vi "sTRING.vi"(6 "angulo":dbl, 8 "Valor del voltaje":dbl, 9 "cadena entrada":string, 10 "Orden":T1(array[ring]), 11 "arreglo opciones":bool[](array[boolean])=[FALSE, FALSE, FALSE, FALSE]) -> (2 "String":string)   [LabVIEW 2016]
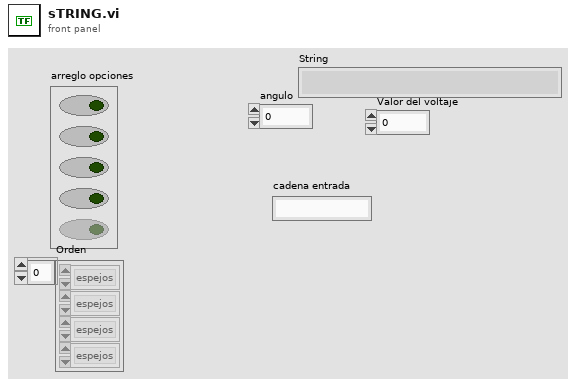
[diagram p1: front panel]
types:
  T1 = enum16{"espejos", "polarizador", "voltaje", "potenciometro y lockin", "CCD"}[]
  T2 = enum16{"espejos", "polarizador", "voltaje", "potenciometro y lockin", "CCD"}
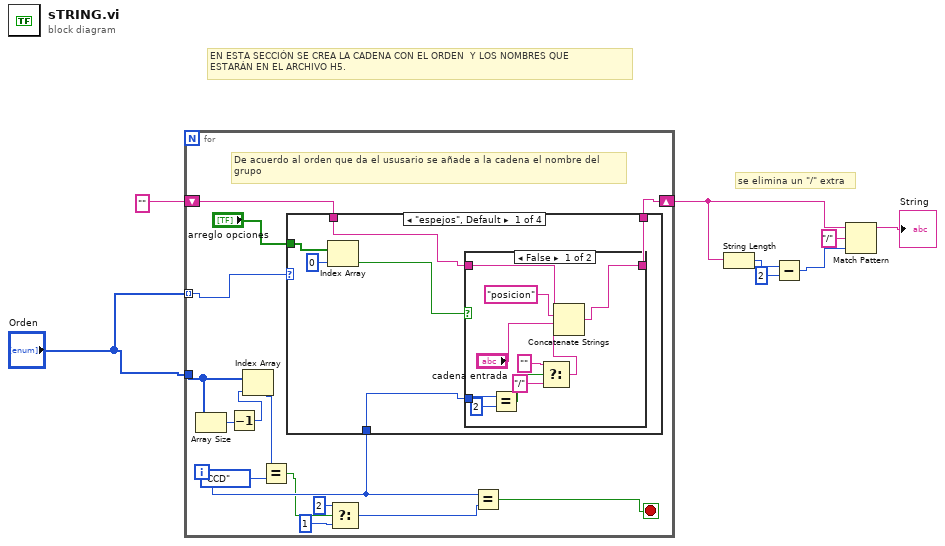
[diagram p0: block diagram]
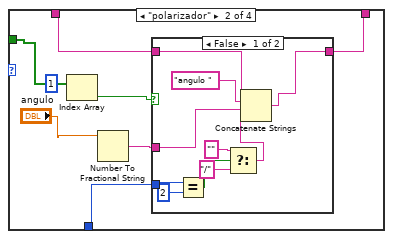
[diagram p3: hidden frame]
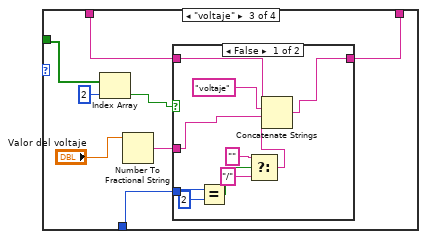
[diagram p5: hidden frame]
diagram:
  # "se elimina un \"/\" extra"
  # "EN ESTA SECCIÓN SE CREA LA CADENA CON EL ORDEN  Y LOS NOMBRES QUE \nESTARÁN EN EL ARCHIVO H5."
  n1 = for {
    tunnel: "Orden" -> [w22] mode=indexing
    shift-right: [w19] -> w5
    shift-left: "" -> [w20]
    tunnel: "Orden" -> [w11]
    i -> [w18]
    stop <- w23 stop-if-true
    # "De acuerdo al orden que da el ususario se añade a la cadena el nombre del\ngrupo"
    n2 = Array Size(array=w11) -> (size(s)=w10:i32)
    n3 = Decrement(x=w10) -> (x-1=w9:i32)
    n4 = Index Array(array=w11, index=w9) -> (element=w17:T2)
    n5 = Equal?(x=w17, y=T2."CCD") -> (x = y?=w13:bool)
    n6 = case shown="\"espejos\", Default" w22 {
      tunnel: "arreglo opciones" -> [w29 w45 w62 _]
      tunnel: w20 -> [w26 w47 w67 w79]
      tunnel: [w25 w43 w66 w79] -> w19
      tunnel: w18 -> [w24 w48 w65 _]
      frame "espejos", Default {
        n7 = Index Array(array=w29, index=0) -> (element=w27:bool)
        n8 = case shown="False" w27 {
          tunnel: w26 -> [w37 w40]
          tunnel: [w36 w40] -> w25
          tunnel: w24 -> [w35 _]
          frame False {
            n9 = Equal?(x=w35, y=2) -> (x = y?=w33:bool)
            n10 = Select(t="", s=w33, f="/") -> (s? t:f=w32:string)
            n11 = Concatenate Strings(w37, "posicion", "cadena entrada", w32) -> (w36:string)
          }
          frame True {
          }
        }
      }
      frame "polarizador" {
        n12 = Index Array(array=w45, index=1) -> (element=w46:bool)
        n13 = Number To Fractional String(number="angulo") -> (F-format string=w44:string)  [unwired: 3 in]
        n14 = case shown="False" w46 {
          tunnel: w47 -> [w57 w59]
          tunnel: [w56 w59] -> w43
          tunnel: w48 -> [w55 _]
          tunnel: w44 -> [w49 _]
          frame False {
            n15 = Equal?(x=w55, y=2) -> (x = y?=w53:bool)
            n16 = Select(t="", s=w53, f="/") -> (s? t:f=w52:string)
            n17 = Concatenate Strings(w57, "angulo ", w49, w52) -> (w56:string)
          }
          frame True {
          }
        }
      }
      frame "voltaje" {
        n18 = Index Array(array=w62, index=2) -> (element=w60:bool)
        n19 = Number To Fractional String(number="Valor del voltaje") -> (F-format string=w64:string)  [unwired: 3 in]
        n20 = case shown="False" w60 {
          tunnel: w67 -> [w76 w78]
          tunnel: [w75 w78] -> w66
          tunnel: w65 -> [w74 _]
          tunnel: w64 -> [w68 _]
          frame False {
            n21 = Equal?(x=w74, y=2) -> (x = y?=w72:bool)
            n22 = Select(t="", s=w72, f="/") -> (s? t:f=w71:string)
            n23 = Concatenate Strings(w76, "voltaje", w68, w71) -> (w75:string)
          }
          frame True {
          }
        }
      }
      frame "potenciometro y lockin" {
      }
    }
    n24 = Select(t=2, s=w13, f=1 ("y")) -> (s? t:f=w14:i32)
    n25 = Equal?(x=w18, y=w14) -> (x = y?=w23:bool)
  }
  n26 = String Length(string=w5) -> (length=w4:i32)
  n27 = Subtract(x=w4, y=2) -> (x-y=w2:i32)
  n28 = Match Pattern(string=w5, regular expression="/", offset (0)=w2) -> (before substring=→"String":string)  [unwired: 3 out]
